vi "Read Element.vi"(8 "error in (no error)":errorcluster, 11 "TypedRefNum.lvclass in":refnum<class "TypedRefNum.lvclass">) -> (0 "error out":errorcluster, 2 "Element":refnum<vi>, 3 "TypedRefNum.lvclass out":refnum<class "TypedRefNum.lvclass">)   [LabVIEW 2015, in "TypedRefNum.lvclass"]
uses:
  TypedRefNum.lvclass
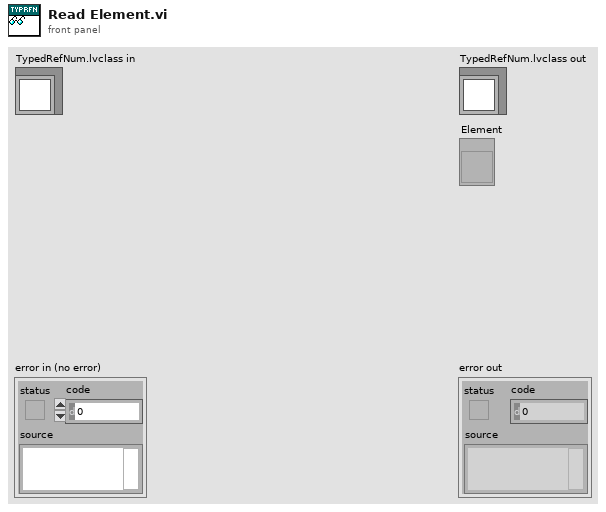
[diagram p1: front panel]
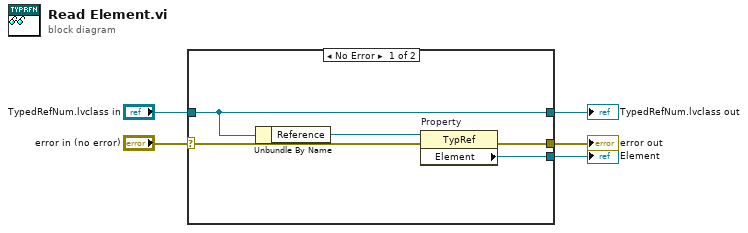
[diagram p0: block diagram]
diagram:
  n1 = case shown="No Error" "error in (no error)" {
    selector: "error in (no error)" -> [w6 w12]
    tunnel: [w9 w12] -> w4
    tunnel: [w8 w11] -> w2
    tunnel: "TypedRefNum.lvclass in" -> [w8 w11]
    tunnel: [w10 _] -> w1
    frame No Error {
      n2 = Unbundle By Name(w8) -> ("Reference"=w7:refnum<vi>)
      n3 = property on="Property" class="TypRef"(reference=w7, error in=w6) -> (error out=w9:errorcluster, "Element"=w10:refnum<vi>)  [unwired: 1 out]
    }
    frame Error {
    }
  }
  "error out" <- w4
  "TypedRefNum.lvclass out" <- w2
  "Element" <- w1
